vi "MW_Close.vi"(8 "error in (no error)":errorcluster, 11 "MW Source Out":T1) -> (0 "error out":errorcluster)   [LabVIEW 2016, in "Microwave Source.lvlib"]
uses:
  Microwave Source.lvlib
  MW_ctl_DeviceHandles..ctl
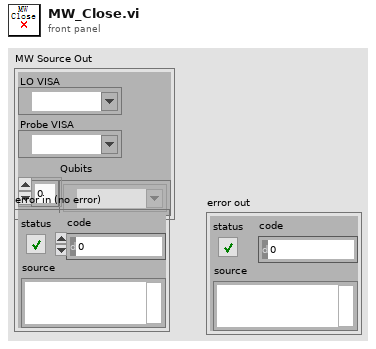
[diagram p1: front panel]
types:
  T1 = typedef "Microwave Source.lvlib/MW_ctl_DeviceHandles..ctl" = cluster{"LO VISA":refnum<visa-resource-name>, "Probe VISA":refnum<visa-resource-name>, "Qubits":refnum<visa-resource-name>[]}
  T2 = typedef "Microwave Source.lvlib/MW_ctl_DeviceType.ctl" = enum16{"R&S", "Other"}
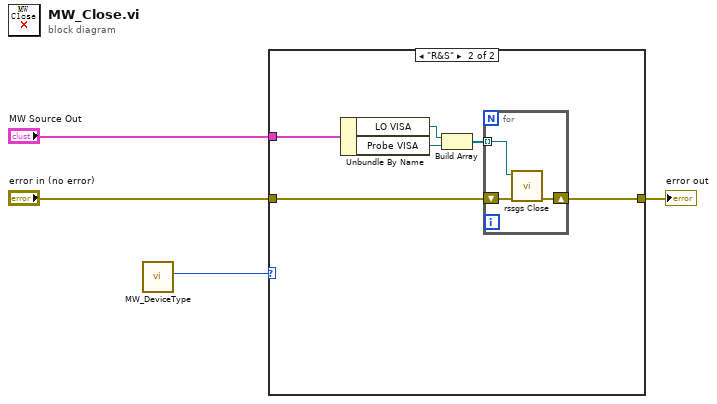
[diagram p0: block diagram]
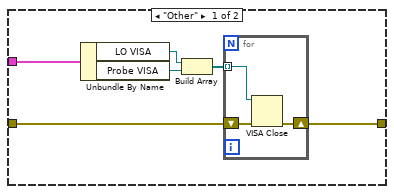
[diagram p2: hidden frame]
diagram:
  n1 = call "MW_DeviceType.vi"() -> ("DeviceType"=w1:T2)  [unwired: 11 in]
  n2 = case shown="\"R&S\"" w1 {
    tunnel: "MW Source Out" -> [w7 w16]
    tunnel: "error in (no error)" -> [w6 w15]
    tunnel: [w5 w14] -> w2
    frame "Other" {
      n3 = Unbundle By Name(w7) -> ("LO VISA"=w8:refnum<visa-resource-name>, "Probe VISA"=w9:refnum<visa-resource-name>)
      n4 = Build Array(w8, w9) -> (w10:refnum<visa-resource-name>[])
      n5 = for {
        shift-right: [w13] -> w5
        shift-left: w6 -> [w12]
        tunnel: w10 -> [w11] mode=indexing
        n6 = VISA Close(VISA resource name=w11, error in (no error)=w12) -> (error out=w13:errorcluster)
      }
    }
    frame "R&S" {
      n7 = Unbundle By Name(w16) -> ("LO VISA"=w17:refnum<visa-resource-name>, "Probe VISA"=w18:refnum<visa-resource-name>)
      n8 = Build Array(w17, w18) -> (w19:refnum<visa-resource-name>[])
      n9 = for {
        shift-right: [w21] -> w14
        shift-left: w15 -> [w22]
        tunnel: w19 -> [w20] mode=indexing
        n10 = call <instrlib>:"rssgs Close.vi"("error in (no error)"=w22, "VISA resource name"=w20) -> ("error out"=w21:errorcluster)  [unwired: 9 in]
      }
    }
  }
  "error out" <- w2
